vi "ScanAction.vi"(8 "error in (no error)":errorcluster caption="entrée d'erreur (pas d'erreur)", 9 "IndicePoint":i32, 10 "Dir":bool, 11 "Tools In":refnum<class "ThorKDC101.lvclass"> caption="DNL_LabVIEW Object in") -> (0 "error out":errorcluster caption="sortie d'erreur", 2 "ScanParsOut":dbl[](array[numeric]), 3 "Tools Out":refnum<class "ThorKDC101.lvclass"> caption="DNL_LabVIEW Object out")   [LabVIEW 2019, in "ThorKDC101.lvclass"]
uses:
  ThorKDC101.lvclass
  C:/Programmes Labview/LabScanV1A/DevicesClass/BaseDevice/BaseDevice.lvclass
  ThorKDC101.lvclass/ThorKDC101.ctl
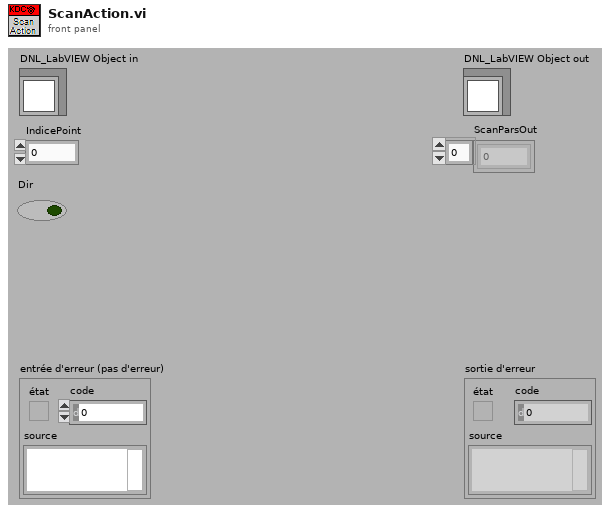
[diagram p1: front panel]
types:
  T1 = typedef "ThorKDC101.lvclass/ThorKDC101_Func.ctl" = enum16{"Position (deg)"}
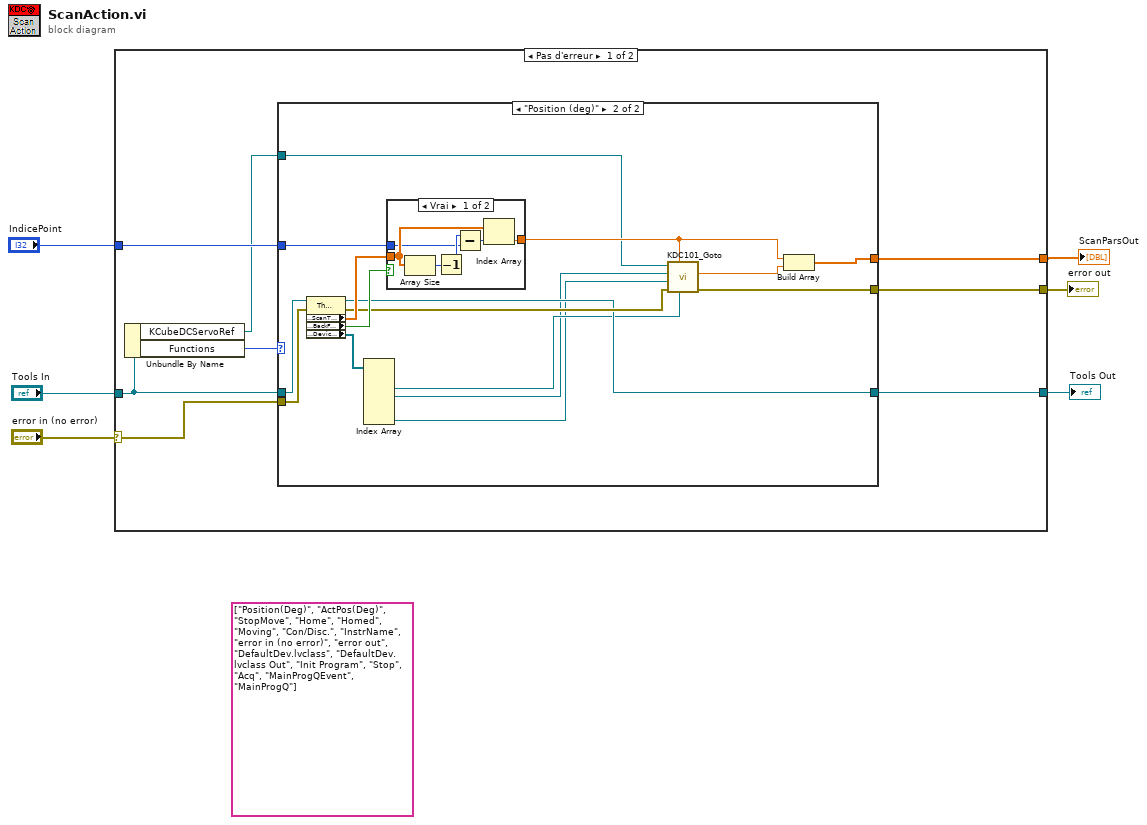
[diagram p0: block diagram]
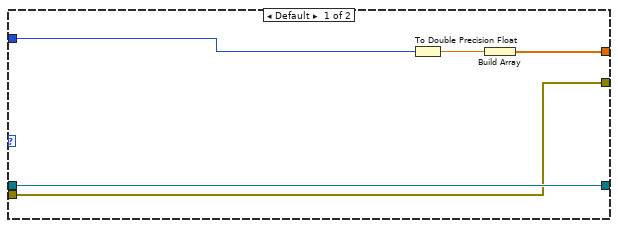
[diagram p2: hidden frame]
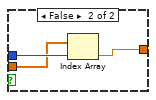
[diagram p3: hidden frame]
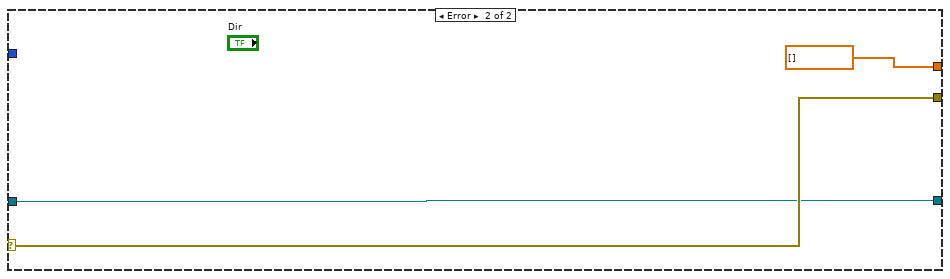
[diagram p4: hidden frame]
diagram:
  (unwired) string[] ["Position(Deg)", "ActPos(Deg)", "StopMove", "Home", "Homed", "Moving", "Con/Disc.", "InstrName", "error in (no error)", "error out", "DefaultDev.lvclass", "DefaultDev.lvclass Out", "Init Program", "Stop", "Acq", "MainProgQEvent", "MainProgQ"] ("ControlsNames")
  n1 = case shown="Pas d'erreur" "error in (no error)" {
    selector: "error in (no error)" -> [w11 w47]
    tunnel: "Tools In" -> [w12 w46]
    tunnel: [w10 dbl[] []] -> w1
    tunnel: [w9 w47] -> w4
    tunnel: [w8 w46] -> w3
    tunnel: "IndicePoint" -> [w13 _]
    frame No Error {
      n2 = Unbundle By Name(w12) -> ("KCubeDCServoRef"=w7:refnum<k24>, "Functions"=w14:T1)
      n3 = case shown="\"Position (deg)\"" w14 {
        tunnel: [w15 w35] -> w10
        tunnel: w13 -> [w19 w30]
        tunnel: [w17 w23] -> w8
        tunnel: w12 -> [w17 w34]
        tunnel: w11 -> [w16 w33]
        tunnel: [w16 w26] -> w9
        tunnel: w7 -> [_ w25]
        frame Default {
          n4 = To Double Precision Float(number=w19) -> (double precision float=w18:dbl)
          n5 = Build Array(w18) -> (w15:dbl[])
        }
        frame "Position (deg)" {
          n6 = property class="ThorKDC101.lvclass"(reference=w34, error in=w33) -> (reference out=w23:refnum<class "ThorKDC101.lvclass">, error out=w24:errorcluster, "Accessor:ScanTable"=w31:dbl[], "Accessor:BackForth"=w32:bool, "Accessor:DeviceCtrl"=w29:refnum<vi>[])
          n7 = Index Array(array=w29) -> (element #2=w22:refnum<vi>, element #3=w21:refnum<vi>, element #6=w20:refnum<vi>)  [unwired: 6 in, 3 out]
          n8 = case shown="Vrai" w32 {
            tunnel: w30 -> [w36 w44]
            tunnel: [w41 w42] -> w28
            tunnel: w31 -> [w40 w43]
            frame True {
              n9 = Array Size(array=w40) -> (size(s)=w39:i32)
              n10 = Decrement(x=w39) -> (x-1=w37:i32)
              n11 = Subtract(x=w37, y=w36) -> (x-y=w38:i32)
              n12 = Index Array(array=w40, index=w38) -> (element=w41:dbl)
            }
            frame False {
              n13 = Index Array(array=w43, index=w44) -> (element=w42:dbl)
            }
          }
          n14 = call <userlib>:"KDC101_Goto.vi"("PositionRef"=w22, "Position(deg)"=w28, "error in (no error)"=w24, "MovingRef"=w20, "StopRef"=w21, "KCubeDCServoRef"=w25) -> ("error out"=w26:errorcluster, "PositionOut(deg)"=w27:dbl)  [unwired: 2 in, 2 out]
          n15 = Build Array(w28, w27) -> (w35:dbl[])
        }
      }
    }
    frame Error {
    }
  }
  "error out" <- w4
  "Tools Out" <- w3
  "ScanParsOut" <- w1
